vi "Create System Status RT FIFO.vi"(8 "error in":errorcluster) -> (0 "error out":errorcluster, 3 "System Status RT FIFO":refnum<k33>)   [LabVIEW 2021, in "RT Main.lvlib"]
uses:
  Libraries/Common RT/Hardware Monitoring.ctl
  RT Main.lvlib
  Libraries/Common RT/Common RT.lvlib
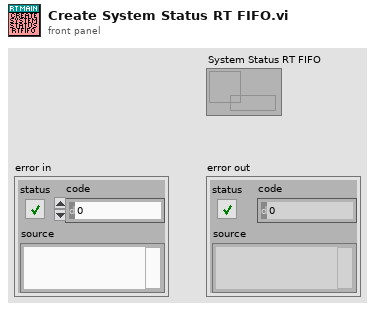
[diagram p1: front panel]
types:
  T1 = typedef "Common RT.lvlib/Hardware Monitoring.ctl" = cluster{"Memory RAM Free (%)":dbl, "Free Flash memory (%)":dbl, "CPU 0 (%)":u32, "CPU 1 (%)":u32}
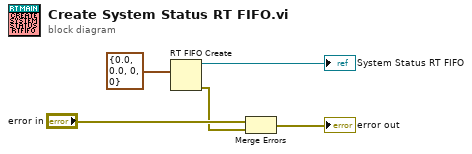
[diagram p0: block diagram]
diagram:
  n1 = RT FIFO Create(1:T1 {"Memory RAM Free (%)"=0.0, "Free Flash memory (%)"=0.0, "CPU 0 (%)"=0, "CPU 1 (%)"=0} ("Hardware Monitoring")) -> (8:→"System Status RT FIFO":refnum<k33>, 11:w2:errorcluster)  [unwired: 7 in, 1 out]
  n2 = Merge Errors("error in", w2) -> (→"error out":errorcluster)
